vi "Test Amplitude Class.vi"(8 "error in (no error)":errorcluster, 11 "TestCase in":refnum<class "Test FGEN.lvclass">) -> (0 "error out":errorcluster, 3 "TestCase out":refnum<class "Test FGEN.lvclass">)   [LabVIEW 2020, in "Test FGEN.lvclass"]
uses:
  Test FGEN.lvclass
  Libraries/FGen/Generador/Generador.lvclass
  Libraries/FGen/GeneradorAmplificado/GeneradorAmplificado.lvclass
  C:/Users/DELL/Documents/GitClones/Labview/IVJoshua2P-/Libraries/FGen/Generador/Generador.lvclass
  Libraries/FGen/Generador/Generador.lvclass/Generador.ctl
  Libraries/FGen/Generador/Set amplitude.vi
  <vilib>/measure/mascope.llb/Amplitude and Levels 1 chan.vi
  <vilib>/addons/_JKI Toolkits/VI Tester/TestCase.llb/TestCase.lvclass
  <vilib>/measure/NI_MAPro.lvlib
  C:/Program Files (x86)/National Instruments/LabVIEW 2020/vi.lib/addons/_JKI Toolkits/VI Tester/TestCase.llb/TestCase.lvclass
panel:
  out "Amplitude":dbl[](array[numeric])
  out "Array":dbl[](array[numeric])
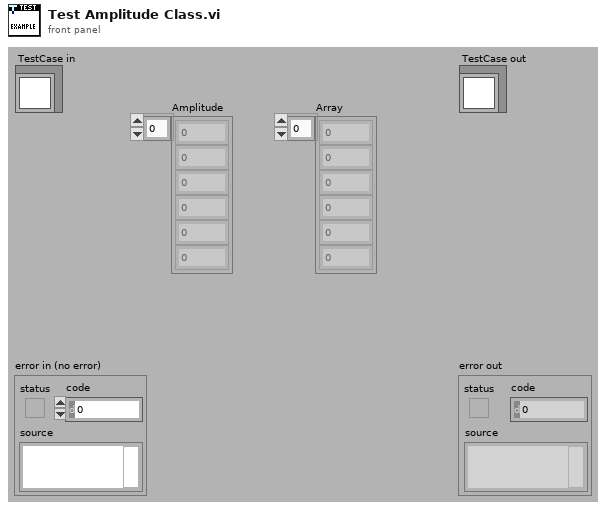
[diagram p1: front panel]
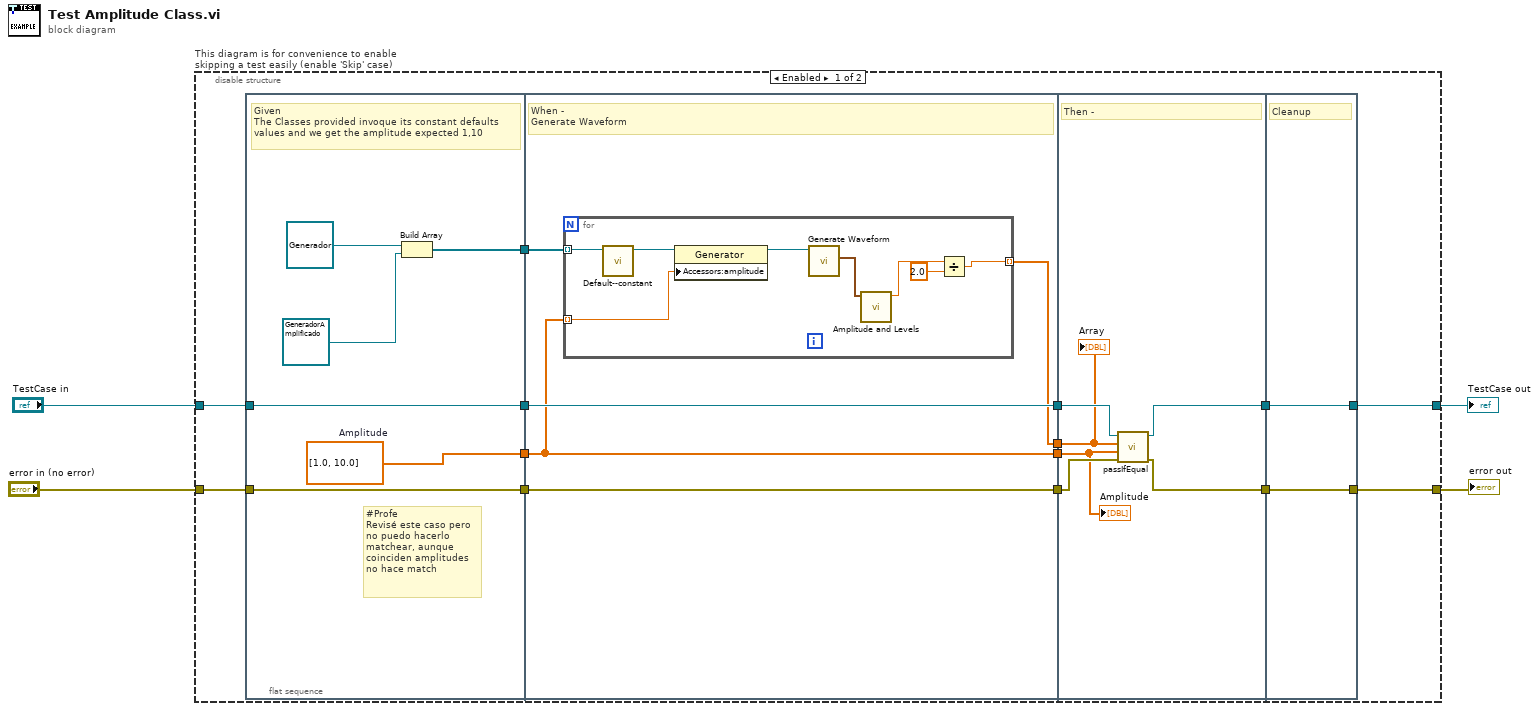
[diagram p0: block diagram]
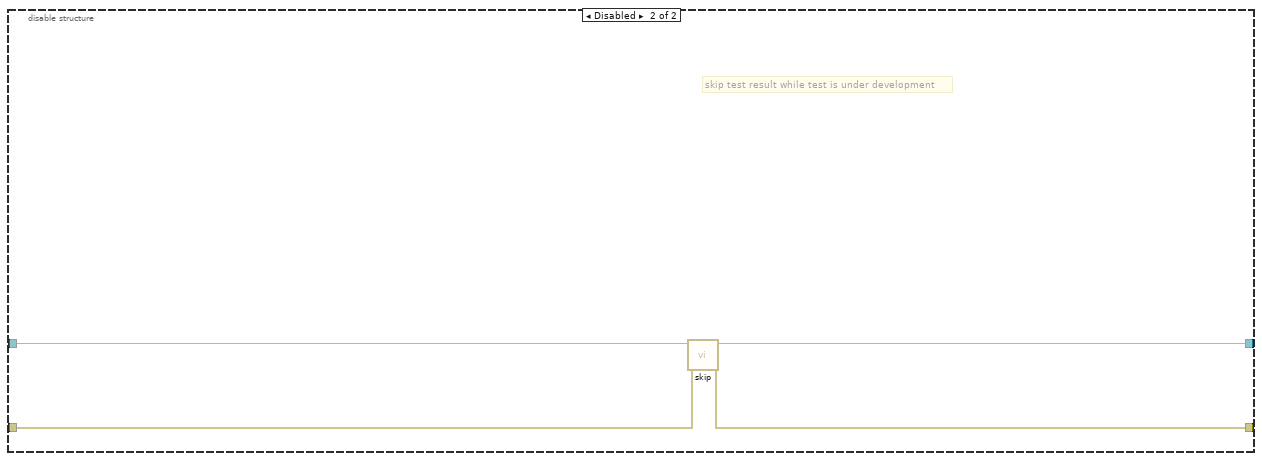
[diagram p2: hidden frame]
diagram:
  n1 = disable-structure "This diagram is for convenience to enable skipping a test easily (enable 'Skip' case)" shown="Enabled" {
    disable-tunnel: "TestCase in" -> [w14 w49]
    disable-tunnel: [w12 w47] -> w1
    disable-tunnel: [w13 w48] -> w3
    disable-tunnel: "error in (no error)" -> [w11 w46]
    frame Enabled {
      n2 = flat-sequence {
        tunnel: w14 -> [w24]
        tunnel: [w24] -> w18
        tunnel: w11 -> [w23]
        tunnel: [w23] -> w9
        tunnel: [w22] -> w7
        tunnel: [w20] -> w5
        tunnel: [w29] -> w17
        tunnel: w18 -> [w29]
        tunnel: [w28] -> w10
        tunnel: w9 -> [w28]
        tunnel: [w27] -> w8
        tunnel: w7 -> [w25]
        tunnel: [w25] -> w6
        tunnel: w5 -> [w26]
        tunnel: [w42] -> w16
        tunnel: [w41] -> w15
        tunnel: w17 -> [w43]
        tunnel: w10 -> [w40]
        tunnel: w8 -> [w39]
        tunnel: w6 -> [w38]
        tunnel: [w44] -> w13
        tunnel: [w45] -> w12
        tunnel: w16 -> [w45]
        tunnel: w15 -> [w44]
        frame #0 {
          w22 = dbl[] [1.0, 10.0]  # Amplitude
          # "#Profe\nRevisé este caso pero\nno puedo hacerlo\nmatchear, aunque\ncoinciden amplitudes\nno hace match"
          # "Given\nThe Classes provided invoque its constant defaults values and we get the amplitude expected 1,10"
          n3 = Build Array(refnum<class "Generador.lvclass"> refnum ("FGen.lvlib:Generator"), refnum<class "GeneradorAmplificado.lvclass"> refnum ("FGen.lvlib:GeneradorAmplificado.lvclass")) -> (w20:refnum<class "Generador.lvclass">[])
        }
        frame #1 {
          # "When -\nGenerate Waveform"
          n4 = for {
            tunnel: [w31] -> w27 mode=indexing
            tunnel: w26 -> [w35] mode=indexing
            tunnel: w25 -> [w32] mode=indexing
            n5 = call-dynamic "Default--constant.vi"("Generator in"=w35) -> ("Generator out"=w34:refnum<class "Generador.lvclass">)  [unwired: 9 in, 1 out]
            n6 = property class="Generator"(reference=w34, "Accessors:amplitude"=w32) -> (reference out=w33:refnum<class "Generador.lvclass">)  [unwired: 1 in, 1 out]
            n7 = call "Generate Waveform.vi"("Generator in"=w33) -> ("Waveform"=w37:waveform(dbl))  [unwired: 8 in, 2 out]
            n8 = call-poly <vilib>:"Amplitude and Levels.vi"("signal in"=w37) -> ("amplitude"=w36:dbl)  [unwired: 7 in, 3 out]
            n9 = Divide(x=w36, y=2.0) -> (x/y=w31:dbl)
          }
        }
        frame #2 {
          # "Then -"
          n10 = call-dynamic "passIfEqual.vi"("error in (no error)"=w40, "y"=w38, "x"=w39, "TestCase in"=w43) -> ("error out"=w41:errorcluster, "TestCase out"=w42:refnum<class "Test FGEN.lvclass">)  [unwired: 6 in]
          "Array" <- w39
          "Amplitude" <- w38
        }
        frame #3 {
          # "Cleanup"
        }
      }
    }
    frame Disabled {
      # "skip test result while test is under development"
      n11 = call <vilib>:"skip.vi"("error in (no error)"=w46, "TestCase in"=w49) -> ("error out"=w48:errorcluster, "TestCase out"=w47:refnum<class "Test FGEN.lvclass">)  [unwired: 8 in]
    }
  }
  "error out" <- w3
  "TestCase out" <- w1
